vi "processFlow.vi"() -> ()   [LabVIEW 2018]
panel:
  out "485Speed":bool=TRUE
  out "manualSpeed":bool=TRUE
  in  "E-Stop 5":bool
  in  "resistance":string
  in  "E-Stop 4":bool
  in  "grade":string
  in  "E-Stop 3":bool
  in  "distance":string
  in  "E-Stop 2":bool
  in  "speed":string
  in  "E-Stop":bool
  out "PowerBoard":bool=TRUE
  out "Controller":bool=TRUE
  in  "type":string
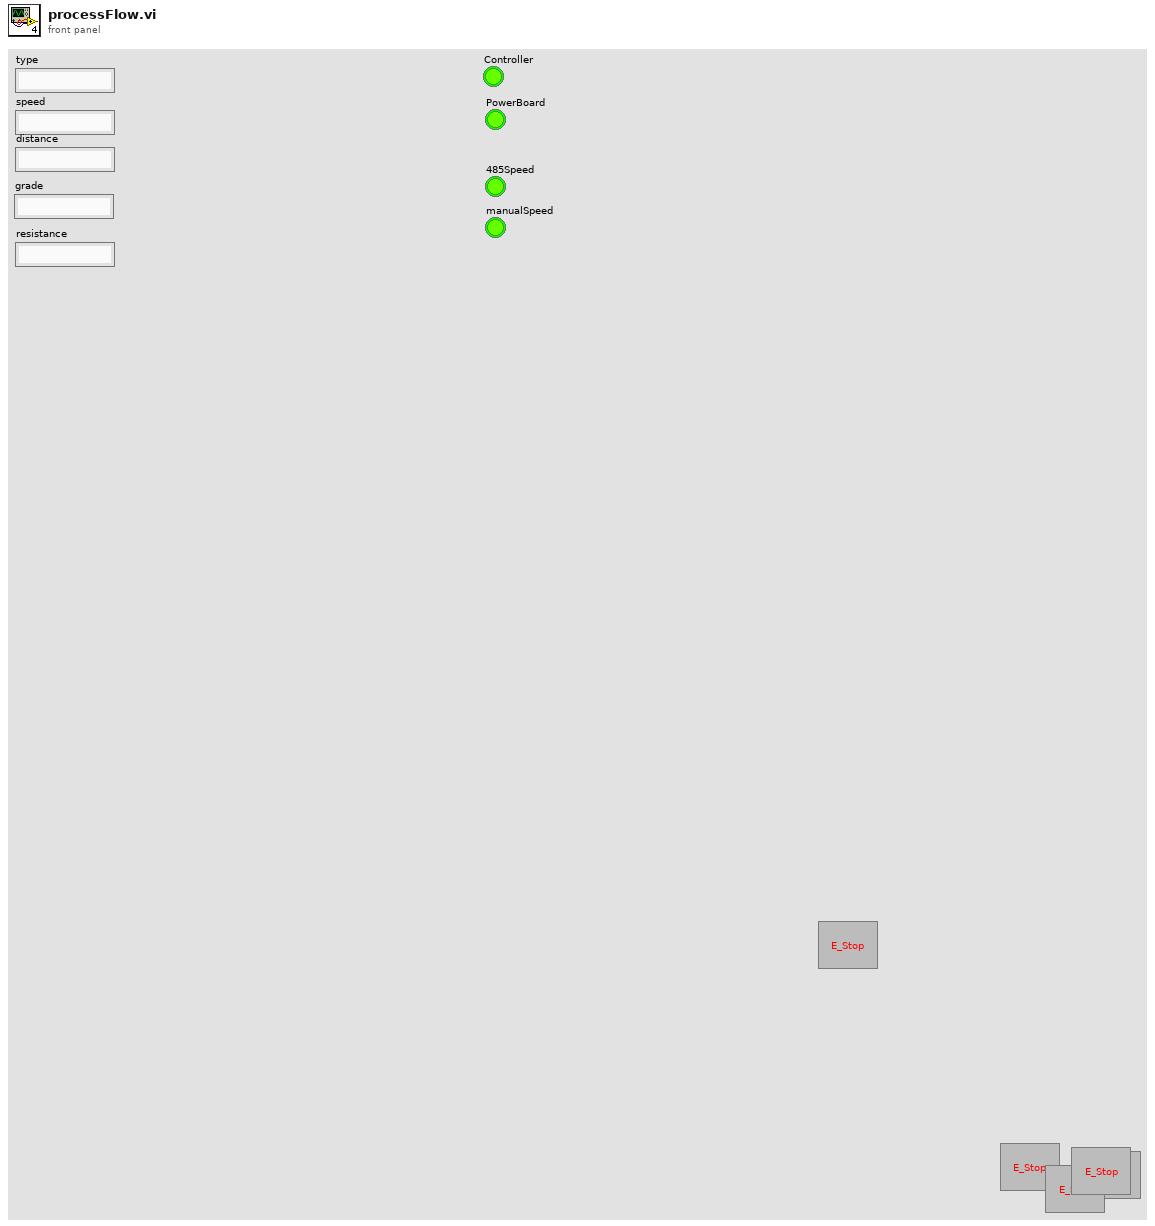
[diagram p1: front panel]
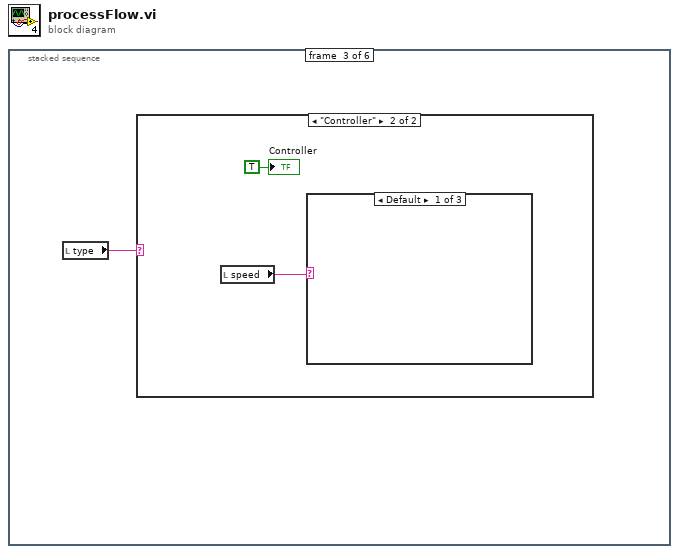
[diagram p0: block diagram]
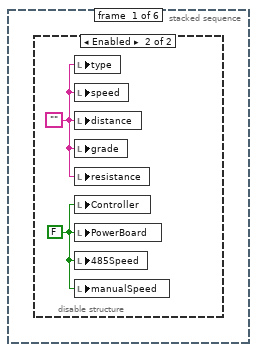
[diagram p2: hidden frame]
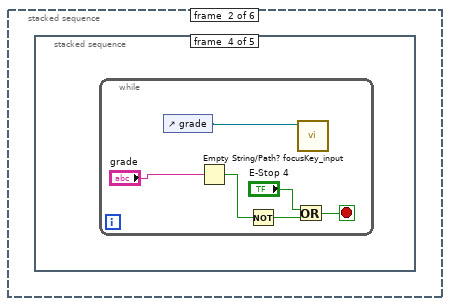
[diagram p4: hidden frame]
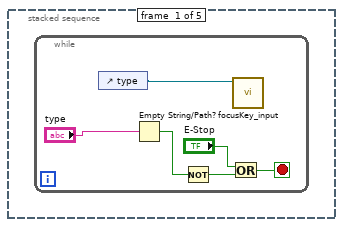
[diagram p5: hidden frame]
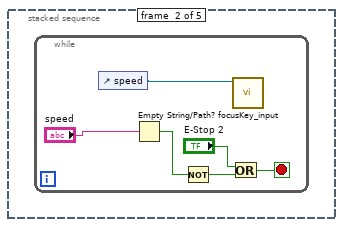
[diagram p6: hidden frame]
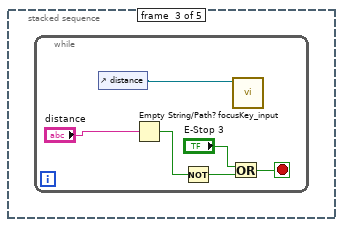
[diagram p7: hidden frame]
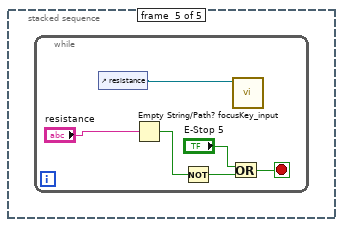
[diagram p8: hidden frame]
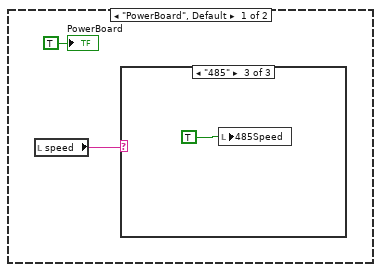
[diagram p9: hidden frame]
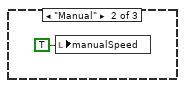
[diagram p11: hidden frame]
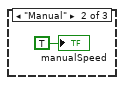
[diagram p12: hidden frame]
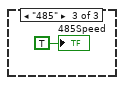
[diagram p13: hidden frame]
diagram:
  n1 = stacked-sequence {
    frame #0 {
      n2 = disable-structure shown="Enabled" {
        frame Disabled {
        }
        frame Enabled {
          w2 = ""
          w1 = FALSE ("Controller")
          n3 = local write "type"(w2) -> ()
          n4 = local write "speed"(w2) -> ()
          n5 = local write "distance"(w2) -> ()
          n6 = local write "grade"(w2) -> ()
          n7 = local write "resistance"(w2) -> ()
          n8 = local write "Controller"(w1) -> ()
          n9 = local write "PowerBoard"(w1) -> ()
          n10 = local write "485Speed"(w1) -> ()
          n11 = local write "manualSpeed"(w1) -> ()
        }
      }
    }
    frame #1 {
      n12 = stacked-sequence {
        frame #0 {
          n13 = while {
            stop <- w6 stop-if-true
            n14 = control-ref of="type"() -> (w3:refnum<vi>)
            n15 = Empty String/Path?(string/path="type") -> (empty?=w8:bool)
            n16 = Not(x=w8) -> (.not. x?=w7:bool)
            n17 = Or(x="E-Stop", y=w7) -> (x .or. y?=w6:bool)
            n18 = call "focusKey_input.vi"("reference"=w3) -> ()  [unwired: 10 in, 1 out]
          }
        }
        frame #1 {
          n19 = while {
            stop <- w12 stop-if-true
            n20 = control-ref of="speed"() -> (w9:refnum<vi>)
            n21 = Empty String/Path?(string/path="speed") -> (empty?=w14:bool)
            n22 = Not(x=w14) -> (.not. x?=w13:bool)
            n23 = Or(x="E-Stop 2", y=w13) -> (x .or. y?=w12:bool)
            n24 = call "focusKey_input.vi"("reference"=w9) -> ()  [unwired: 10 in, 1 out]
          }
        }
        frame #2 {
          n25 = while {
            stop <- w18 stop-if-true
            n26 = control-ref of="distance"() -> (w15:refnum<vi>)
            n27 = Empty String/Path?(string/path="distance") -> (empty?=w20:bool)
            n28 = Not(x=w20) -> (.not. x?=w19:bool)
            n29 = Or(x="E-Stop 3", y=w19) -> (x .or. y?=w18:bool)
            n30 = call "focusKey_input.vi"("reference"=w15) -> ()  [unwired: 10 in, 1 out]
          }
        }
        frame #3 {
          n31 = while {
            stop <- w24 stop-if-true
            n32 = control-ref of="grade"() -> (w21:refnum<vi>)
            n33 = Empty String/Path?(string/path="grade") -> (empty?=w26:bool)
            n34 = Not(x=w26) -> (.not. x?=w25:bool)
            n35 = Or(x="E-Stop 4", y=w25) -> (x .or. y?=w24:bool)
            n36 = call "focusKey_input.vi"("reference"=w21) -> ()  [unwired: 10 in, 1 out]
          }
        }
        frame #4 {
          n37 = while {
            stop <- w30 stop-if-true
            n38 = control-ref of="resistance"() -> (w27:refnum<vi>)
            n39 = Empty String/Path?(string/path="resistance") -> (empty?=w32:bool)
            n40 = Not(x=w32) -> (.not. x?=w31:bool)
            n41 = Or(x="E-Stop 5", y=w31) -> (x .or. y?=w30:bool)
            n42 = call "focusKey_input.vi"("reference"=w27) -> ()  [unwired: 10 in, 1 out]
          }
        }
      }
    }
    frame #2 {
      n43 = local read "type"() -> (w33:string)
      n44 = case shown="\"Controller\"" w33 {
        frame "PowerBoard", Default {
          n45 = local read "speed"() -> (w34:string)
          n46 = case shown="\"485\"" w34 {
            frame Default {
            }
            frame "Manual" {
              n47 = local write "manualSpeed"(TRUE) -> ()
            }
            frame "485" {
              n48 = local write "485Speed"(TRUE) -> ()
            }
          }
          "PowerBoard" <- TRUE
        }
        frame "Controller" {
          n49 = local read "speed"() -> (w38:string)
          n50 = case shown="Default" w38 {
            frame Default {
            }
            frame "Manual" {
              "manualSpeed" <- TRUE
            }
            frame "485" {
              "485Speed" <- TRUE
            }
          }
          "Controller" <- TRUE
        }
      }
    }
    frame #3 {
    }
    frame #4 {
    }
    frame #5 {
    }
  }
